vi "Waveform Generation.vi"(11 "Cluster":T1) -> (1 "Output Y Values":dbl[](array[numeric]), 3 "Waveform":waveform(dbl))   [LabVIEW 2014]
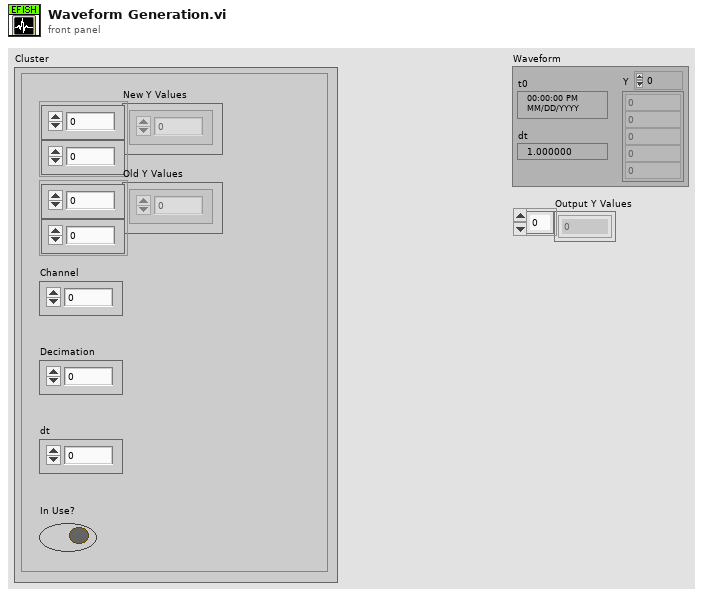
[diagram p1: front panel]
types:
  T1 = cluster{"New Y Values":dbl[][], "Old Y Values":dbl[][], "Channel":i8, "Decimation":i16, "dt":dbl, "In Use?":bool}
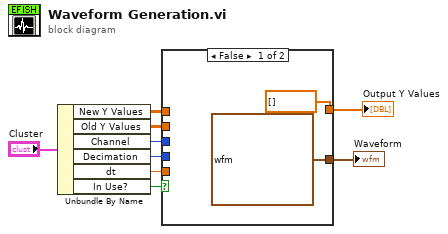
[diagram p0: block diagram]
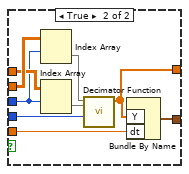
[diagram p2: hidden frame]
diagram:
  n1 = Unbundle By Name("Cluster") -> ("New Y Values"=w8:dbl[][], "Old Y Values"=w7:dbl[][], "Channel"=w6:i8, "Decimation"=w5:i16, "dt"=w3:dbl, "In Use?"=w4:bool)
  n2 = case shown="False" w4 {
    tunnel: w7 -> [_ w20]
    tunnel: w8 -> [_ w19]
    tunnel: w6 -> [_ w18]
    tunnel: w5 -> [_ w17]
    tunnel: w3 -> [_ w14]
    tunnel: [waveform(dbl) {"t0"=timestamp(0 s since 1904-01-01), "dt"=1.0, "Y"=[]} w13] -> w2
    tunnel: [dbl[] [] ("Output Y Values") w12] -> w1
    frame False {
    }
    frame True {
      n3 = Index Array(array=w20, index (row)=w18) -> (element=w16:dbl[])  [unwired: 1 in]
      n4 = Index Array(array=w19, index (row)=w18) -> (element=w15:dbl[])  [unwired: 1 in]
      n5 = call "Decimator Function.vi"("Decimation #"=w17, "Input Y values New"=w15, "Input Y values Old"=w16) -> ("Output Y Values"=w12:dbl[])  [unwired: 8 in]
      n6 = Bundle By Name("Y"=w12, "dt"=w14) -> (w13:waveform(dbl))  [unwired: 1 in]
    }
  }
  "Waveform" <- w2
  "Output Y Values" <- w1
